vi "Check Size.vi"(7 "source vi name":string, 8 "error in (no error)":errorcluster, 10 "required size":u64 format="%08x bytes", 11 "Pointer in":refnum<class "Pointer.lvclass">) -> (0 "error out":errorcluster, 2 "required size out":u64 format="%08x bytes", 3 "Pointer out":refnum<class "Pointer.lvclass">)   [LabVIEW 2027, in "Memory Manager.lvlib" / "Pointer.lvclass"]
uses:
  Pointer.lvclass
  Out of Bounds.vi
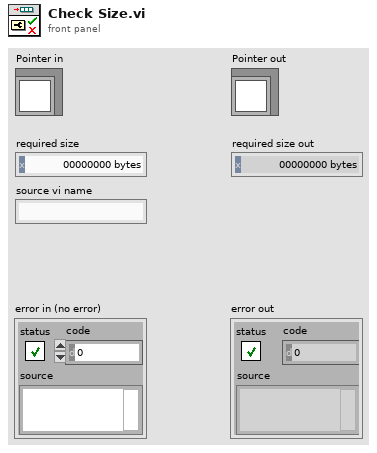
[diagram p1: front panel]
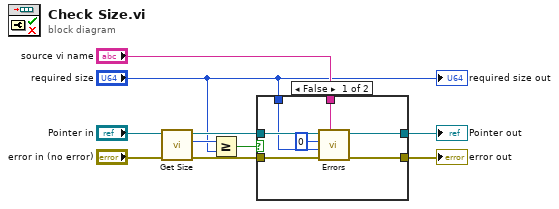
[diagram p0: block diagram]
diagram:
  n1 = call "Get Size.vi"("Pointer in"="Pointer in") -> ("size"=w7:u64, "Pointer out"=w4:refnum<class "Pointer.lvclass">)  [unwired: 9 in]
  n2 = Greater Or Equal?(x=w7, y="required size") -> (x >= y?=w5:bool)
  n3 = case shown="False" w5 {
    tunnel: w4 -> [w16 w17]
    tunnel: "error in (no error)" -> [w14 w18]
    tunnel: [w13 w18] -> w9
    tunnel: [w15 w17] -> w8
    tunnel: "required size" -> [w12 _]
    tunnel: "source vi name" -> [w11 _]
    frame False {
      n4 = call-poly "Errors.vi"("error source vi name"=w11, "error in (no error)"=w14, "size"=w12, "offset"=u64 0, "Pointer in"=w16) -> ("error out"=w13:errorcluster, "Pointer out"=w15:refnum<class "Pointer.lvclass">)  [unwired: 5 in]
    }
    frame True {
    }
  }
  "error out" <- w9
  "Pointer out" <- w8
  "required size out" <- "required size"
